vi "Write Temperature Control.lvclass.vi"(10 "Temperature Control.lvclass":refnum<class "Temperature Control.lvclass">, 11 "Test Framework in":refnum<class "Test Framework.lvclass">) -> (3 "Test Framework out":refnum<class "Test Framework.lvclass">)   [LabVIEW 2020, in "Test Framework.lvclass"]
uses:
  Test Framework.lvclass
  Instruments/Temperature Control/Temperature Control.lvclass
  Test Framework.lvclass/Test Framework.ctl
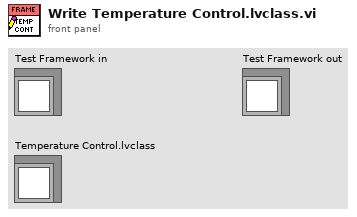
[diagram p1: front panel]
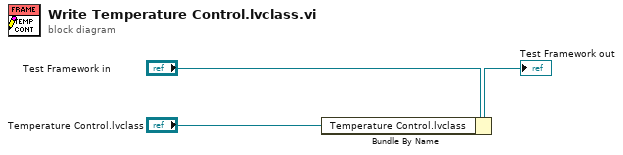
[diagram p0: block diagram]
diagram:
  n1 = Bundle By Name(cluster="Test Framework in", "Temperature Control.lvclass"="Temperature Control.lvclass") -> (→"Test Framework out":refnum<class "Test Framework.lvclass">)
